vi "CalcdeltaV.vi"(4 "Correction":dbl[][](array[numeric])=[[450.0, 0.0, 0.0], [460.0, 0.0, 0.0], [480.0, 2.0, 1.0], [500.0, 0.0, 2.0], [520.0, -2.0, 3.0], [540.0, -2.0, 2.0], [560.0, -7.0, 4.0], [580.0, -12.0, 4.0], [600.0, -19.0, 6.0], [620.0, -23.0, 7.0], [640.0, -26.0, 8.0], [660.0, -28.0, 9.0], [680.0, -28.0, 9.0], [700.0, -24.0, 8.0], [720.0, -24.0, 8.0], [740.0, -20.0, 8.0], [760.0, -20.0, 8.0], [780.0, -20.0, 8.0]], 5 "nm0":dbl, 6 "nm in":dbl, 7 "Volts/pixel y":dbl, 8 "Volts/pixel  x":dbl) -> (0 "DeltaVy":dbl, 1 "Delta Pix y":dbl, 2 "delta pix x":dbl, 3 "DeltaVx":dbl)   [LabVIEW 2013]
panel:
  # "Included delta pix for testing"
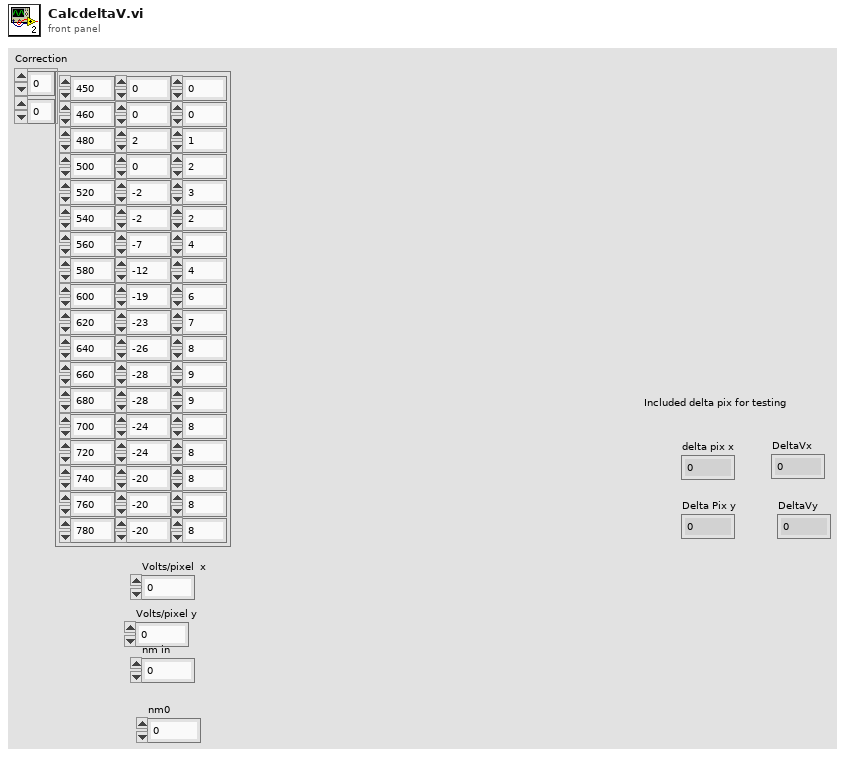
[diagram p1: front panel]
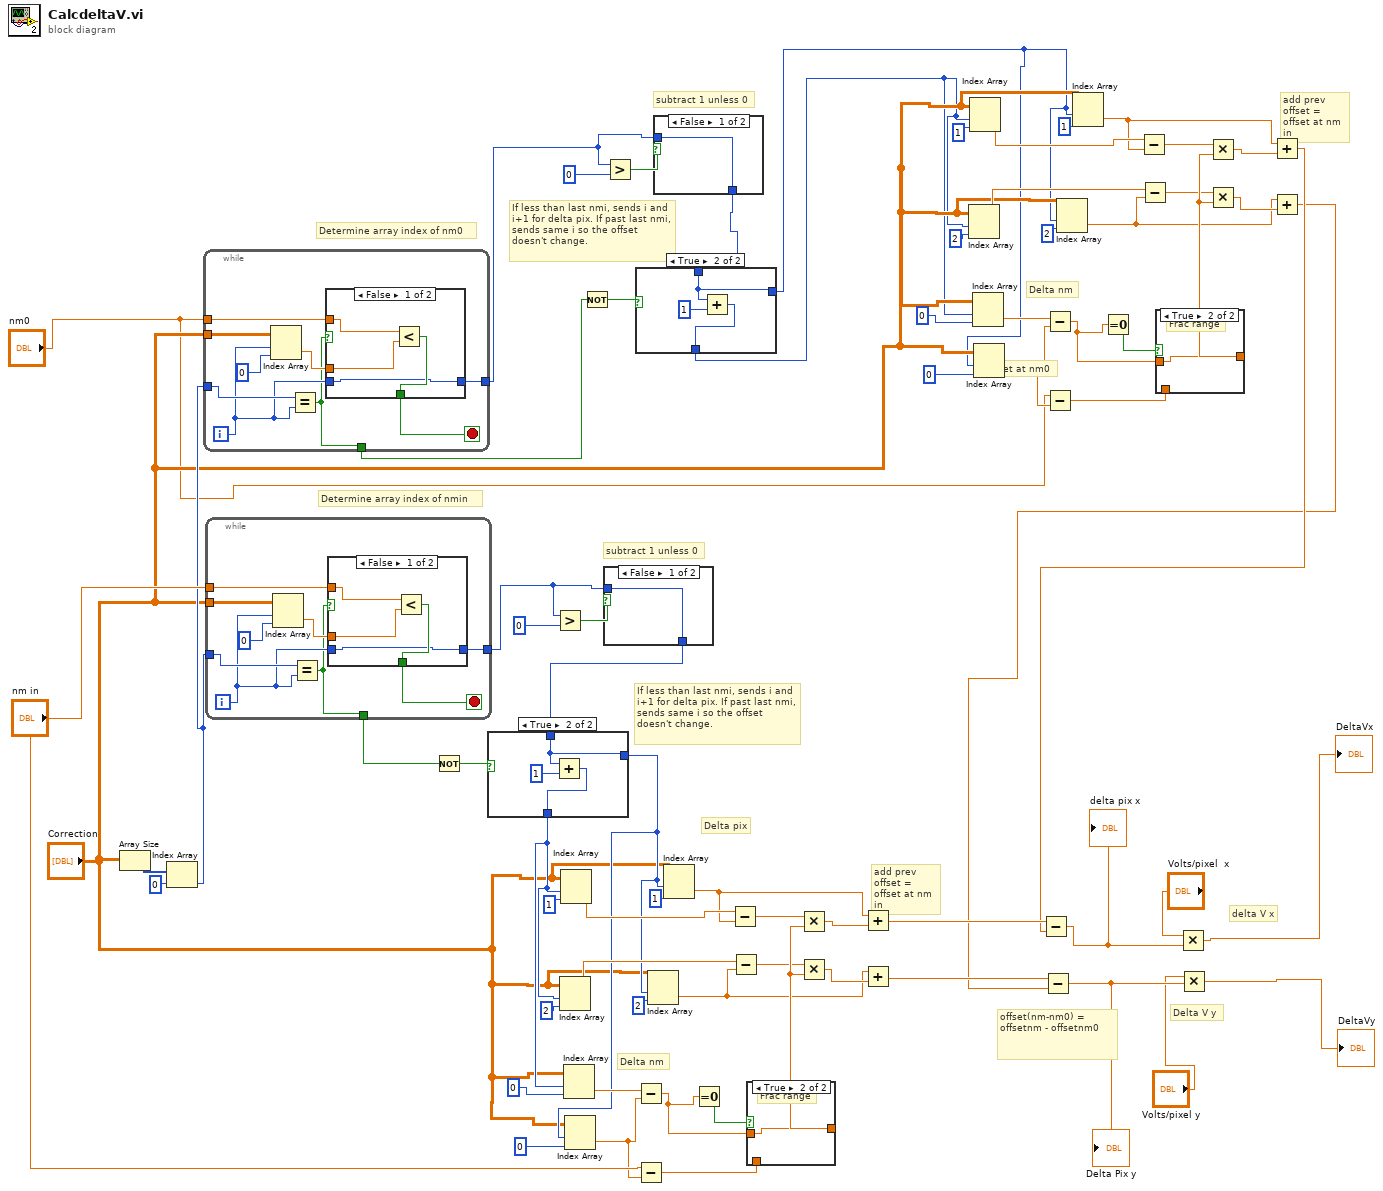
[diagram p0: block diagram]
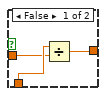
[diagram p3: hidden frame]
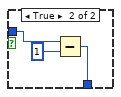
[diagram p4: hidden frame]
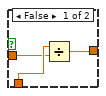
[diagram p6: hidden frame]
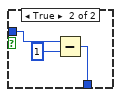
[diagram p8: hidden frame]
diagram:
  # "If less than last nmi, sends i and i+1 for delta pix. If past last nmi, sends same i so the offset doesn't change."
  # "add prev offset = offset at nm in"
  # "Delta nm"
  # "offset(nm-nm0) = offsetnm - offsetnm0"
  # "offset at nm0"
  # "subtract 1 unless 0"
  # "Determine array index of nm0"
  # "If less than last nmi, sends i and i+1 for delta pix. If past last nmi, sends same i so the offset doesn't change."
  # "delta V x"
  # "add prev offset = offset at nm in"
  # "subtract 1 unless 0"
  # "Determine array index of nmin"
  # "Delta nm"
  # "Delta V y"
  # "Delta pix"
  n1 = Array Size(array="Correction") -> (size(s)=w66:i32[])
  n2 = Index Array(array=w66, index=0) -> (element=w40:i32)
  n3 = while {
    tunnel: w40 -> [w80]
    tunnel: "nm0" -> [w77]
    tunnel: [w79] -> w37
    tunnel: "Correction" -> [w75]
    tunnel: [w73] -> w9
    i -> [w74]
    stop <- w78 stop-if-true
    n4 = Index Array(array=w75, index (row)=w74, index (col)=0 ("disabled index (col)")) -> (element=w76:dbl)
    n5 = Equal?(x=w80, y=w74) -> (x = y?=w73:bool)
    n6 = case shown="False" w73 {
      selector: w73 -> [_ w86]
      tunnel: w74 -> [w82 w87]
      tunnel: [w82 w87] -> w79
      tunnel: [w83 w86] -> w78
      tunnel: w77 -> [w85 _]
      tunnel: w76 -> [w84 _]
      frame False {
        n7 = Less?(x=w85, y=w84) -> (x < y?=w83:bool)
      }
      frame True {
      }
    }
  }
  n8 = while {
    tunnel: w40 -> [w95]
    tunnel: "nm in" -> [w92]
    tunnel: [w94] -> w61
    tunnel: "Correction" -> [w90]
    tunnel: [w88] -> w47
    i -> [w89]
    stop <- w93 stop-if-true
    n9 = Index Array(array=w90, index (row)=w89, index (col)=0 ("disabled index (col)")) -> (element=w91:dbl)
    n10 = Equal?(x=w95, y=w89) -> (x = y?=w88:bool)
    n11 = case shown="False" w88 {
      selector: w88 -> [_ w101]
      tunnel: w89 -> [w97 w102]
      tunnel: [w97 w102] -> w94
      tunnel: [w98 w101] -> w93
      tunnel: w92 -> [w100 _]
      tunnel: w91 -> [w99 _]
      frame False {
        n12 = Less?(x=w100, y=w99) -> (x < y?=w98:bool)
      }
      frame True {
      }
    }
  }
  n13 = Not(x=w47) -> (.not. x?=w46:bool)
  n14 = Greater?(x=w61, y=0) -> (0:w62:bool)
  n15 = Not(x=w9) -> (.not. x?=w10:bool)
  n16 = case shown="False" w62 {
    tunnel: w61 -> [w103 w106]
    tunnel: [w103 w104] -> w48
    frame False {
    }
    frame True {
      n17 = Subtract(x=w106, y=1) -> (x-y=w104:i32)
    }
  }
  n18 = case shown="True" w46 {
    tunnel: [w107 w109] -> w45
    tunnel: w48 -> [w107 w108]
    tunnel: [w107 w108] -> w44
    frame False {
    }
    frame True {
      n19 = Add(x=w108, y=1) -> (x+y=w109:i32)
    }
  }
  n20 = Index Array(array="Correction", index (row)=w45, index (col)=2 ("index")) -> (element=w56:dbl)
  n21 = Index Array(array="Correction", index (row)=w45, index (col)=1 ("index")) -> (element=w57:dbl)
  n22 = Index Array(array="Correction", index (row)=w45, index (col)=0 ("index")) -> (element=w71:dbl)
  n23 = Index Array(array="Correction", index (row)=w44, index (col)=0 ("index")) -> (element=w41:dbl)
  n24 = Greater?(x=w37, y=0) -> (0:w39:bool)
  n25 = Subtract(x=w71, y=w41) -> (x-y=w42:dbl)
  n26 = Subtract(x="nm in", y=w41) -> (x-y=w60:dbl)
  n27 = Index Array(array="Correction", index (row)=w44, index (col)=2) -> (element=w50:dbl)
  n28 = case shown="False" w39 {
    tunnel: w37 -> [w111 w114]
    tunnel: [w111 w112] -> w7
    frame False {
    }
    frame True {
      n29 = Subtract(x=w114, y=1) -> (x-y=w112:i32)
    }
  }
  n30 = case shown="True" w10 {
    tunnel: [w115 w117] -> w5
    tunnel: w7 -> [w115 w116]
    tunnel: [w115 w116] -> w6
    frame False {
    }
    frame True {
      n31 = Add(x=w116, y=1) -> (x+y=w117:i32)
    }
  }
  n32 = Index Array(array="Correction", index (row)=w44, index (col)=1) -> (element=w49:dbl)
  n33 = Equal To 0?(x=w42) -> (x = 0?=w43:bool)
  n34 = Subtract(x=w57, y=w49) -> (x-y=w54:dbl)
  n35 = Subtract(x=w56, y=w50) -> (x-y=w53:dbl)
  n36 = case shown="True" w43 {
    tunnel: w60 -> [w121 _]
    tunnel: w42 -> [w120 w122]
    tunnel: [w119 w122] -> w55
    frame False {
      n37 = Divide(x=w121, y=w120) -> (x/y=w119:dbl)
    }
    frame True {
      # "Frac range"
    }
  }
  n38 = Multiply(x=w54, y=w55) -> (x*y=w52:dbl)
  n39 = Multiply(x=w53, y=w55) -> (x*y=w51:dbl)
  n40 = Add(x=w49, y=w52) -> (x+y=w36:dbl)
  n41 = Add(x=w50, y=w51) -> (x+y=w35:dbl)
  n42 = Index Array(array="Correction", index (row)=w5, index (col)=2 ("index")) -> (element=w21:dbl)
  n43 = Index Array(array="Correction", index (row)=w5, index (col)=1 ("index")) -> (element=w22:dbl)
  n44 = Index Array(array="Correction", index (row)=w5, index (col)=0 ("index")) -> (element=w30:dbl)
  n45 = Index Array(array="Correction", index (row)=w6, index (col)=0 ("index")) -> (element=w11:dbl)
  n46 = Subtract(x=w30, y=w11) -> (x-y=w12:dbl)
  n47 = Subtract(x="nm0", y=w11) -> (x-y=w25:dbl)
  n48 = Index Array(array="Correction", index (row)=w6, index (col)=2) -> (element=w15:dbl)
  n49 = Index Array(array="Correction", index (row)=w6, index (col)=1) -> (element=w14:dbl)
  n50 = Equal To 0?(x=w12) -> (x = 0?=w13:bool)
  n51 = Subtract(x=w22, y=w14) -> (x-y=w19:dbl)
  n52 = Subtract(x=w21, y=w15) -> (x-y=w18:dbl)
  n53 = case shown="True" w13 {
    tunnel: w25 -> [w125 _]
    tunnel: w12 -> [w124 w126]
    tunnel: [w123 w126] -> w20
    frame False {
      n54 = Divide(x=w125, y=w124) -> (x/y=w123:dbl)
    }
    frame True {
      # "Frac range"
    }
  }
  n55 = Multiply(x=w19, y=w20) -> (x*y=w17:dbl)
  n56 = Multiply(x=w18, y=w20) -> (x*y=w16:dbl)
  n57 = Add(x=w14, y=w17) -> (x+y=w3:dbl)
  n58 = Subtract(x=w36, y=w3) -> (x-y=w34:dbl)
  "delta pix x" <- w34
  n59 = Multiply(x="Volts/pixel  x", y=w34) -> (x*y=→"DeltaVx":dbl)
  n60 = Add(x=w15, y=w16) -> (x+y=w2:dbl)
  n61 = Subtract(x=w35, y=w2) -> (x-y=w33:dbl)
  "Delta Pix y" <- w33
  n62 = Multiply(x="Volts/pixel y", y=w33) -> (x*y=→"DeltaVy":dbl)
